vi "Dashboard Main.vi"() -> ()   [LabVIEW 2018]
uses:
  <vilib>/Utility/miscctls.llb/LVRowAndColumnTypeDef.ctl
  <vilib>/event_ctls.llb/eventvkey.ctl
  <vilib>/Rock Robotics/Network Tables/NT Read Boolean.vi
  <vilib>/Rock Robotics/Network Tables/NT Write Boolean.vi
  <vilib>/Rock Robotics/Network Tables/NT Read Numeric Array.vi
  <vilib>/Rock Robotics/WPI/Dashboard/WPI_DashboardLogging Global.vi
panel:
  in  "Camera Settings Right":T1={"Frame Rate"=30, "Compression"=30, "Size"=1, "DB Camera Config"=FALSE} {"Frame Rate" scale=1.0..30.0; "Compression" scale=100.0..-1.0; "Size" items=["640x480", "320x240", "160x120"]}
  in  "Camera Name Right":string(combo)="No Camera Selection"
  out "Camera Perf":string
  in  "Camera Settings":T1={"Frame Rate"=30, "Compression"=30, "Size"=1, "DB Camera Config"=FALSE} {"Frame Rate" scale=1.0..30.0; "Compression" scale=100.0..-1.0; "Size" items=["640x480", "320x240", "160x120"]}
  in  "TCP":refnum<k5>
  in  "Rec Mode":enum32{"Stop", "Record", "Playback"}(radio)
  out "Image Message":string="Timeout in Camera Communications"
  in  "Dashboard Tab":T2(tab)
  in  "Auto Side":bool
  out "Limelight Target State":bool
  out "Hatch Open":bool
  out "Hatch Extend":bool
  out "Cargo Piston":bool
  in  "Zero Yaw":bool
  out "Yaw":dbl
  out "Cont Yaw":dbl
  out "LowerLimit":bool
  out "UpperLimit":bool
  out "HAB Retracting limit":bool
  out "HAB Extending limit":bool
  in  "Select Auto":string(combo)="Select Autonomous ..."
  out "NT Connection":bool
  out "Mode":T3(ring)=enum."Auto Disabled"
  out "Right Camera Perf":cluster{"Bandwidth (Mbps)":dbl, "FPS":dbl}
  out "Lift Auto Position":u16(ring) items=["Cargo 1", "Hatch 1", "Cargo 2", "Hatch 2", "Cargo 3", "Hatch 3"]
  out "CargoLimit":bool
  out "Wheel Rates":T4
  out "Wheel Angles":T4
  out "Y-Velocity":dbl
  out "X-Velocity":dbl
  out "Wheel Positions":T4
  out "Lift Height":dbl
  out "Graph":cluster{cluster{"X":dbl, "Y":dbl}[]}[](graph)
  out "Positions":cluster{"X":dbl, "Y":dbl}
  out "Tree":string(tree)
  in  "Test Slider":dbl(slide) scale=0.0..100.0 scale format="%#_3g"
  in  "On/Off":bool caption="Solenoid"
  in  "Test Name":u16(ring) items=["Select the test to run..."]
  in  "Test Tree":string(tree)
  in  "Motor":cluster{"Value":dbl, "Enable":bool} {"Value" scale=-1.0..1.0 scale format="%#_3g"}
  out "Progress":T5 {"Test Progress" scale=0.0..100.0}
  in  "Rev/Fwd":cluster{"Forward":bool, "Reverse":bool}
  in  "Test Ring":u16(ring) items=["Monochrome", "Color"]
  in  "CheckList":i32(listbox)
  out "Cmd Status":string
  in  "Execute Command":bool
  in  "Command Params":string[][](table)
  in  "Command Selection":i32(listbox)
  out "Camera Image":T6(plugin-control)
  in  "Camera Name":string(combo)="No Camera Selection"
  # "HW"
  # "HW"
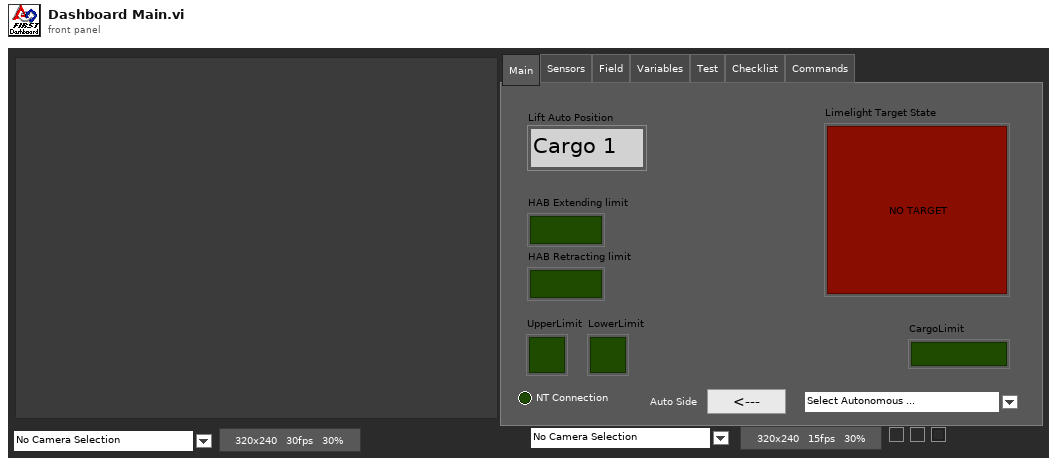
[diagram p1: front panel]
types:
  T1 = cluster{"Frame Rate":i32, "Compression":i32, "Size":u16, "DB Camera Config":bool}
  T2 = enum32{"Main", "Sensors", "Field", "Variables", "Test", "Checklist", "Commands"}
  T3 = enum8{"Tele-Op Disabled", "Tele-Op Enabled", "Auto Disabled", "Auto Enabled", "Test Disabled", "Test Enabled", "Disconnected", "No Code", "E-Stop"}
  T4 = cluster{"FrontLeft":dbl, "FrontRight":dbl, "BackLeft":dbl, "BackRight":dbl}
  T5 = cluster{"Test Progress":u8, "Test Progress Text":string}
  T6 = typedef "IMAQ Image.ctl" = refnum<image>
  T7 = cluster{"Save Path":path, "Interval (s)":dbl, "Keep":i32}
  T8 = enum32{"Drive", "Camera", "Basic", "Custom", "Test", "Commands", "Checklist", "Variables"}
  T9 = typedef "Image Type" = u32
  T10 = cluster{"IDs":cluster{"RPC field ID":u16, "Unique ID":u16}, "String":string}
  T11 = cluster{"Error Strings":string, "Disable Counts":cluster{u16, u16}, "Rail Faults":cluster{u16, u16, u16}, "Robot IP":string, "DB Mode":u8, "Event Info":cluster{"Name":string, "Type":u8, "Number":u16, "Replay":u8}}
  T12 = cluster{"Storage":cluster{"Disk Free":u64, "RAM Block":u32, "RAM free":u32}, "CPU Utilization":cluster{"CPU % ISR":sgl, "CPU % Time Crit":sgl, "CPU % Timed Str":sgl, "CPU % High":sgl, "CPU % Above":sgl, "CPU % Normal":sgl, "CPU % Low":sgl}, "CAN":cluster{"% Bus Utilization":sgl, "Bus Off Cnt":u32, "TX_FIFO Full Cnt":u32, "Receive Error Cnt":u8, "Transmit Error Cnt":u8}, "HID":cluster{"HID Outputs":u32, "Rumble Low":u16, "Rumble High":u16}[]}
  T13 = cluster{"Status bits":cluster{"Test Mode":bool, "Autonomous":bool, "Enabled":bool, "Code Start":bool, "Brownout":bool, "Reserved 2":bool, "Reserved 3":bool, "E-Stop":bool}, "Code Trace":cluster{"Disabled":bool, "TeleOp":bool, "Auto":bool, "Test":bool}, "Controller Type":enum16{"unknown", "cRIO", "roboRio"}, "Code?":enum16{"unknown", "noCode", "code"}, "Battery V":dbl}
  T14 = cluster{"Control Bits":cluster{"TestMode":bool, "Autonomous":bool, "Enabled":bool, "FMS Present":bool, bool, bool, bool, "E-Stop":bool}, "Team Station ":u8, "Countdown":sgl, "Joystick Values":cluster{"Axes":dbl[], "Buttons":bool[], "POVs":i16[]}[]}
  T15 = cluster{"Numeric":dbl, "Numeric":dbl, "Numeric":dbl, "Numeric":dbl}
  T16 = cluster{"Global Rectangle":i32[], "Contours":cluster{"Contour Type":u32, "ROI Type":u32, "Points":i32[]}[]}
  T17 = cluster{"Camera Name":string, string, "Saved DB Images Info":cluster{"Save Path":path, "Interval (s)":dbl, "Keep":i32}}
  T18 = cluster{"Camera Name Right":string, string, "Saved DB Images Info":cluster{"Save Path":path, "Interval (s)":dbl, "Keep":i32}}
  T19 = cluster{"Operation":enum16{"Update", "Clear"}, "Color Box":u32}[]
  T20 = typedef "eventvkey.ctl" = enum16{"ASCII", "Enter", "Return", "Shift", "Ctrl", "Alt", "Cmd", "Opt", "Caps", "NumLock", "Clear", "Break", "Up", "Down", "Left", "Right", "Insert", "Delete", "Home", "End", "PageUp", "PageDown", "Escape", "Help", "Pause", "ScrollLock", "F1", "F2", "F3", "F4", "F5", "F6", "F7", "F8", "F9", "F10", "F11", "F12", "F13", "F14", "F15", "F16", "F17", "F18", "F19", "F20", "F21", "F22", "F23", "F24", "Play", "VolumeUp", "VolumeDown", "Mute", "Two Byte Char"}
  T21 = cluster{"Operation":enum16{"Update", "Clear"}, "Color Box":u32}
  T22 = typedef "LVRowAndColumnTypeDef.ctl" = cluster{"Row":i32, "Column":i32}
  T23 = cluster{"Shift":bool, "Ctrl":bool, "Alt":bool, "Cmd":bool, "Opt":bool}
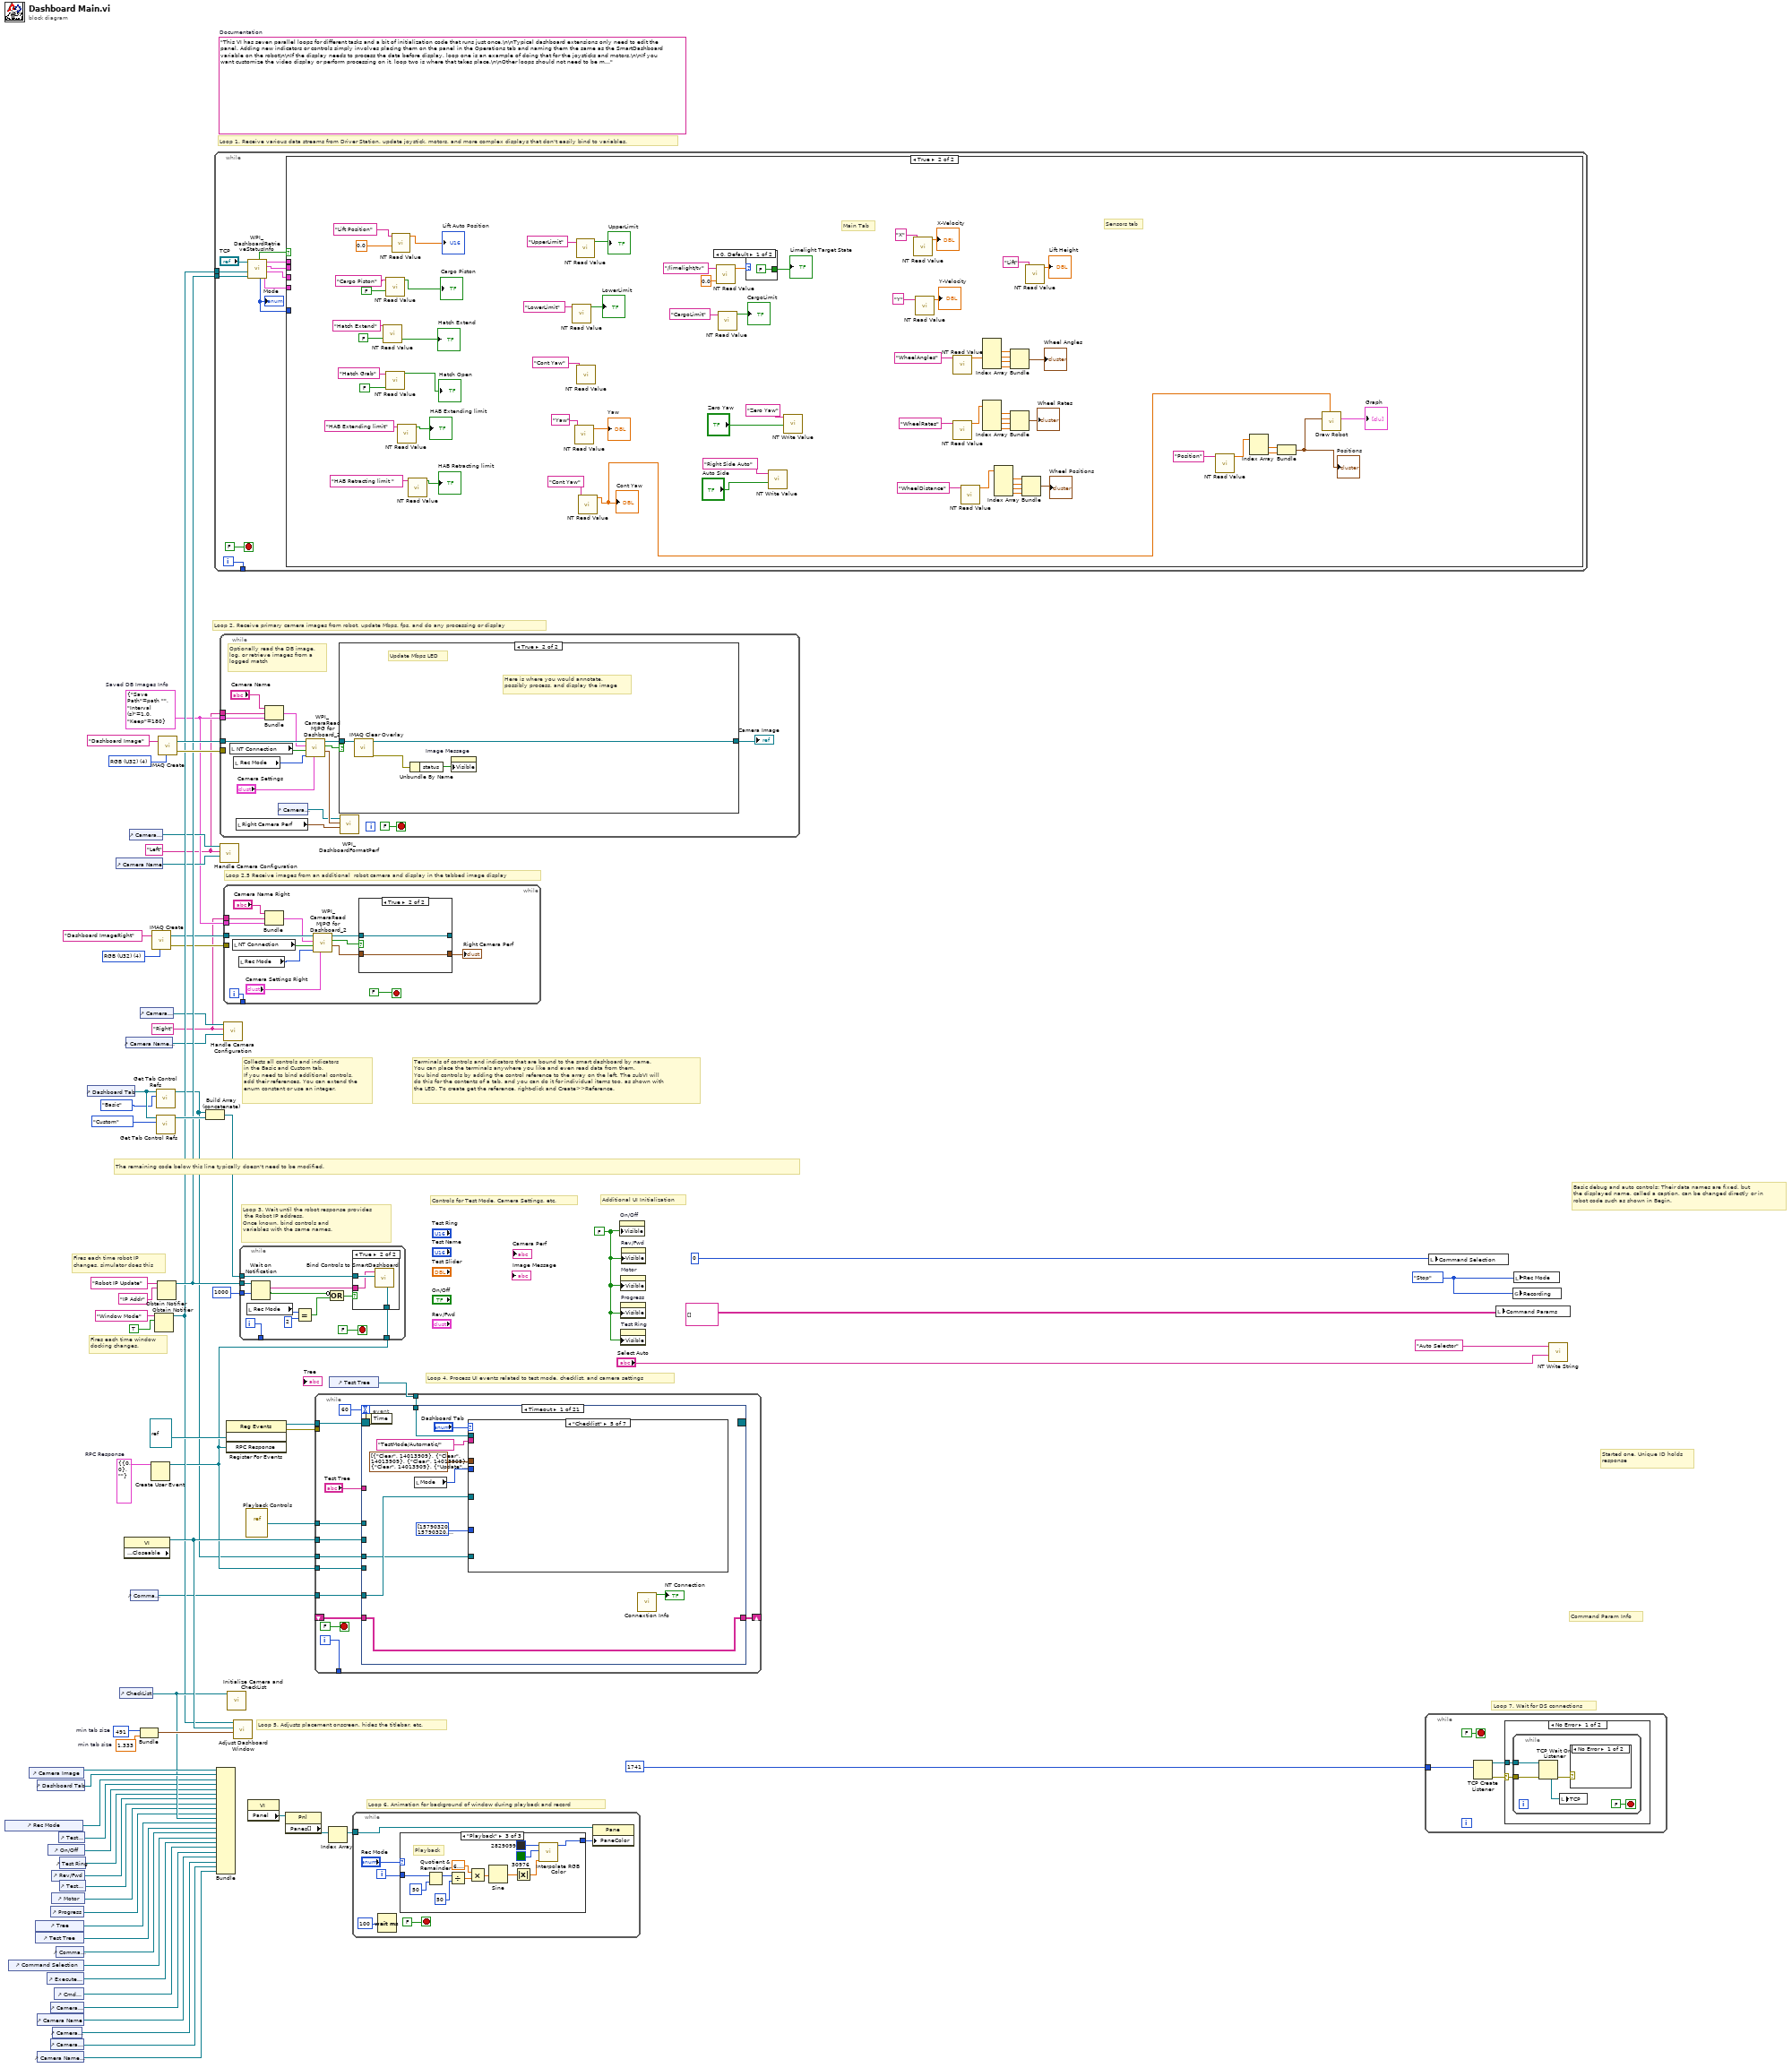
[diagram p0: block diagram]
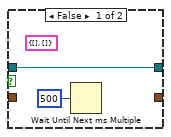
[diagram p2: hidden frame]
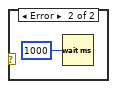
[diagram p3: hidden frame]
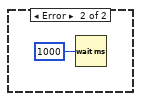
[diagram p4: hidden frame]
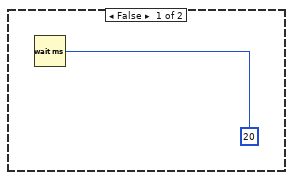
[diagram p5: hidden frame]
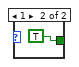
[diagram p6: hidden frame]
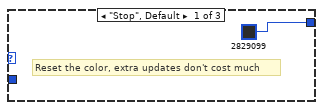
[diagram p7: hidden frame]
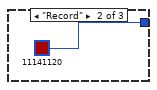
[diagram p8: hidden frame]
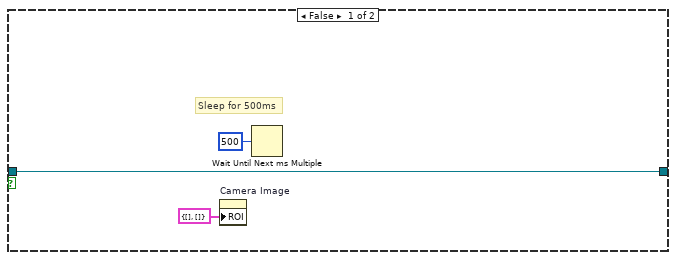
[diagram p10: hidden frame]
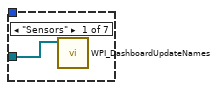
[diagram p11: hidden frame]
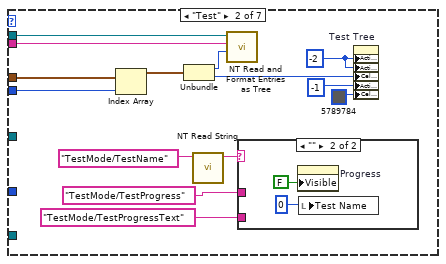
[diagram p12: hidden frame]
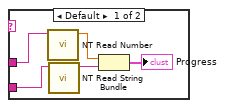
[diagram p13: hidden frame]
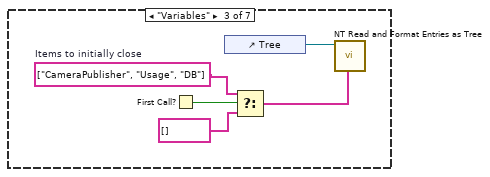
[diagram p14: hidden frame]
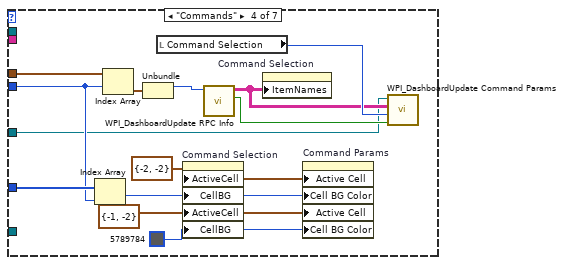
[diagram p15: hidden frame]
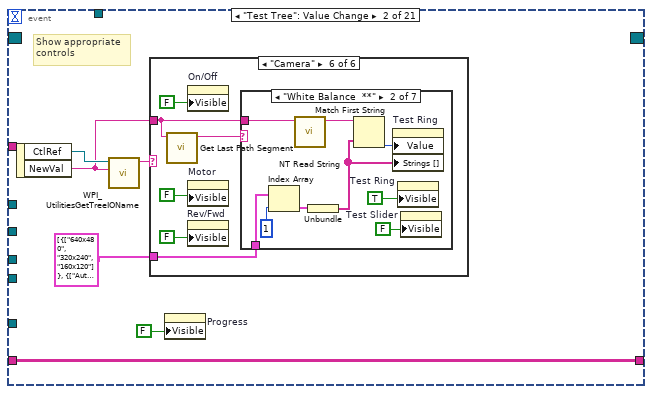
[diagram p18: hidden frame]
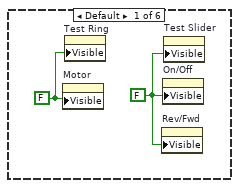
[diagram p19: hidden frame]
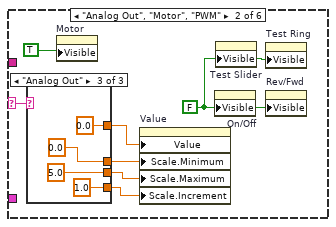
[diagram p20: hidden frame]
diagram:
  w3 = T7 {"Save Path"=path "", "Interval (s)"=1.0, "Keep"=180}  # Saved DB Images Info
  w2 = "Right"
  w1 = "Left"
  w12 = T9 4 items=["Grayscale (U8)", "Grayscale (I16)", "Grayscale (SGL)", "Complex (CSG)", "RGB (U32)", "HSL (U32)", "RGB (U64)"] ("Image Type")
  w28 = T10 {"IDs"={"RPC field ID"=0, "Unique ID"=0}, "String"=""}  # RPC Response
  w48 = 491  # min tab size
  w47 = 1.333  # min tab size
  w55 = enum32{"Stop", "Record", "Playback"}."Stop" ("Rec Mode")
  w34 = FALSE ("Visible")
  (unwired) "This VI has seven parallel loops for different tasks and a bit of initialization code that runs just once.\n\nTypical dashboard extensions only need to edit the panel. Adding new indicators or controls simply involves placing them on the panel in the Operations tab and naming them the same as the SmartDashboard variable on the robot\n\nIf the display needs to process the data before display, loop one is an example of doing that for the joysticks and motors.\n\nIf you want customize the video display or perform processing on it, loop two is where that takes place.\n\nOther loops should not need to be modified. They are pretty standard, and document the task they perform."  # Documentation
  w72 = T9 4 items=["Grayscale (U8)", "Grayscale (I16)", "Grayscale (SGL)", "Complex (CSG)", "RGB (U32)", "HSL (U32)", "RGB (U64)"] ("Image Type")
  # "Loop 2.5 Receive images from an additional  robot camera and display in the tabbed image display"
  # "Command Param Info"
  # "Started one, Unique ID holds\nresponse"
  # "Loop 7. Wait for DS connections"
  # "Basic debug and auto controls: Their data names are fixed, but\nthe displayed name, called a caption, can be changed directly or in\nrobot code such as shown in Begin."
  # "Controls for Test Mode, Camera Settings, etc."
  # "Additional UI Initialization"
  # "Loop 6. Animation for background of window during playback and record"
  # "Fires each time robot IP\nchanges, simulator does this"
  # "Fires each time window\ndocking changes."
  # "Collects all controls and indicators\nin the Basic and Custom tab.\nIf you need to bind additional controls,\nadd their references. You can extend the\nenum constant or use an integer."
  # "The remaining code below this line typically doesn't need to be modified."
  # "Loop 4. Process UI events related to test mode, checklist, and camera settings"
  # "Terminals of controls and indicators that are bound to the smart dashboard by name.\nYou can place the terminals anywhere you like and even read data from them.\nYou bind controls by adding the control reference to the array on the left. The subVI will\ndo this for the contents of a tab, and you can do it for individual items too, as shown with\nthe LED. To create get the reference, right-click and Create>>Reference."
  # "Loop 3. Wait until the robot response provides\n the Robot IP address.\nOnce known, bind controls and\nvariables with the same names."
  # "Loop 5. Adjusts placement onscreen, hides the titlebar, etc."
  # "Loop 1. Receive various data streams from Driver Station, update joystick, motors, and more complex displays that don't easily bind to variables."
  # "Loop 2. Receive primary camera images from robot, update Mbps, fps, and do any processing or display"
  n1 = control-ref of="Rec Mode"() -> (w40:refnum<vi>)
  n2 = control-ref of="Command Selection"() -> (w27:refnum<vi>)
  n3 = control-ref of="Camera Image"() -> (w50:refnum<vi>)
  n4 = control-ref of="Tree"() -> (w44:refnum<vi>)
  n5 = control-ref of="Test Tree"() -> (w43:refnum<vi>)
  n6 = control-ref of="Dashboard Tab"() -> (w49:refnum<vi>)
  n7 = control-ref of="Camera Name"() -> (w18:refnum<vi>)
  n8 = control-ref of="Camera Name Right"() -> (w6:refnum<vi>)
  n9 = control-ref of="Execute Command"() -> (w29:refnum<vi>)
  n10 = control-ref of="On/Off"() -> (w38:refnum<vi>)
  n11 = control-ref of="Progress"() -> (w35:refnum<vi>)
  n12 = control-ref of="Camera Settings"() -> (w19:refnum<vi>)
  n13 = control-ref of="Camera Settings Right"() -> (w7:refnum<vi>)
  n14 = control-ref of="Rev/Fwd"() -> (w36:refnum<vi>)
  n15 = control-ref of="Motor"() -> (w41:refnum<vi>)
  n16 = control-ref of="Camera Perf"() -> (w17:refnum<vi>)
  n17 = control-ref of="Cmd Status"() -> (w23:refnum<vi>)
  n18 = control-ref of="Command Params"() -> (w30:refnum<vi>)
  n19 = control-ref of="Test Slider"() -> (w39:refnum<vi>)
  n20 = control-ref of="Test Ring"() -> (w37:refnum<vi>)
  n21 = control-ref of="Test Name"() -> (w42:refnum<vi>)
  n22 = control-ref of="Dashboard Tab"() -> (w53:refnum<vi>)
  n23 = control-ref of="Camera Name"() -> (w20:refnum<vi>)
  n24 = control-ref of="CheckList"() -> (w45:refnum<vi>)
  n25 = property class="VI" props=["Front Panel.Closeable"]() -> (reference out=w54:refnum<vi>)  [unwired: 2 in, 2 out]
  n26 = control-ref of="Camera Name Right"() -> (w8:refnum<vi>)
  n27 = control-ref of="Camera Settings"() -> (w21:refnum<vi>)
  n28 = control-ref of="Command Params"() -> (w22:refnum<vi>)
  n29 = control-ref of="Camera Settings Right"() -> (w9:refnum<vi>)
  n30 = Bundle("min tab size"=w48, "min tab size"=w47) -> (w46:cluster{"min tab size":i32, "min tab size":dbl})  [unwired: 1 in]
  n31 = Create User Event(user event datatype=w28) -> (user event=w24:refnum<user-event>)  [unwired: 1 in, 1 out]
  n32 = call "IMAQ Create"("Image Name"="Dashboard ImageRight", "Image Type"=w12) -> ("New Image"=w11:T6, "error out"=w10:errorcluster)  [unwired: 2 in, 1 out]
  n33 = Obtain Notifier(name (unnamed)="Window Mode", notification data type=TRUE) -> (notifier out=w32:refnum<notifier>)  [unwired: 2 in, 2 out]
  n34 = call <vilib>:"Get Tab Control Refs.vi"("Page Index"=T8."Basic" ("Dashboard Tab"), "TabControl in"=w53) -> ("ControlsOnPage"=w16:refnum<vi>[])  [unwired: 9 in]
  n35 = call <vilib>:"Get Tab Control Refs.vi"("Page Index"=T8."Custom" ("Dashboard Tab"), "TabControl in"=w53) -> ("ControlsOnPage"=w52:refnum<vi>[])  [unwired: 9 in]
  n36 = Obtain Notifier(name (unnamed)="Robot IP Update", notification data type="IP Addr" ("name (unnamed)")) -> (notifier out=w33:refnum<notifier>)  [unwired: 2 in, 2 out]
  n37 = call "IMAQ Create"("Image Name"="Dashboard Image", "Image Type"=w72) -> ("New Image"=w70:T6, "error out"=w69:errorcluster)  [unwired: 2 in, 1 out]
  n38 = Build Array (concatenate)(w16, w52) -> (w51:refnum<vi>[])
  n39 = while {
    tunnel: [w82] -> _
    tunnel: w33 -> [w80]
    tunnel: w32 -> [w77]
    i -> [w82]
    stop <- FALSE stop-if-true
    n40 = call <vilib>:"WPI_DashboardRetrieveStatusInfo.vi"("Binding Refnum"=w80, "Window Mode Notifier"=w77, "TCP Cnx"="TCP") -> ("Power and Errors"=w74:T11, "Robot Metrics"=w73:T12, "Status Info"=w75:T13, "Control Info"=w76:T14, "Robot Mode"=w79:T3, "Process?"=w81:bool)  [unwired: 3 in]
    "Mode" <- w79
    n41 = case shown="True" w81 {
      tunnel: w79 -> [_ _]
      tunnel: w76 -> [_ _]
      tunnel: w75 -> [_ _]
      tunnel: w74 -> [_ _]
      tunnel: w73 -> [_ _]
      frame False {
        n42 = Wait (ms)(milliseconds to wait=u32 20) -> ()  [unwired: 1 out]
      }
      frame True {
        # "Sensors tab"
        # "Main Tab"
        n43 = call-poly <vilib>:"NT Read Value.vi"("Default Value"=FALSE, "Name"="Hatch Extend") -> ("Boolean"=→"Hatch Extend":bool)  [unwired: 8 in, 1 out]
        n44 = call-poly <vilib>:"NT Read Value.vi"("Default Value"=FALSE, "Name"="Cargo Piston") -> ("Boolean"=→"Cargo Piston":bool)  [unwired: 8 in, 1 out]
        n45 = call-poly <vilib>:"NT Read Value.vi"("Default Value"=FALSE, "Name"="Hatch Grab") -> ("Boolean"=→"Hatch Open":bool)  [unwired: 8 in, 1 out]
        n46 = call-poly <vilib>:"NT Read Value.vi"("Default Value"=0.0, "Name"="Lift Position") -> ("Numeric"=→"Lift Auto Position":dbl)  [unwired: 8 in, 1 out]
        n47 = call-poly <vilib>:"NT Read Value.vi"("Name"="HAB Extending limit") -> ("Boolean"=→"HAB Extending limit":bool)  [unwired: 9 in, 1 out]
        n48 = call-poly <vilib>:"NT Read Value.vi"("Name"="HAB Retracting limit ") -> ("Boolean"=→"HAB Retracting limit":bool)  [unwired: 9 in, 1 out]
        n49 = call-poly <vilib>:"NT Read Value.vi"("Name"="LowerLimit") -> ("Boolean"=→"LowerLimit":bool)  [unwired: 9 in, 1 out]
        n50 = call-poly <vilib>:"NT Read Value.vi"("Name"="Yaw") -> ("Numeric"=→"Yaw":dbl)  [unwired: 9 in, 1 out]
        n51 = call-poly <vilib>:"NT Read Value.vi"("Name"="UpperLimit") -> ("Boolean"=→"UpperLimit":bool)  [unwired: 9 in, 1 out]
        n52 = call-poly <vilib>:"NT Read Value.vi"("Name"="Cont Yaw") -> ()  [unwired: 9 in, 2 out]
        n53 = call-poly <vilib>:"NT Read Value.vi"("Name"="Cont Yaw") -> ("Numeric"=w85:dbl)  [unwired: 9 in, 1 out]
        "Cont Yaw" <- w85
        n54 = call-poly <vilib>:"NT Read Value.vi"("Default Value"=0.0, "Name"="/limelight/tv") -> ("Numeric"=w120:dbl)  [unwired: 8 in, 1 out]
        n55 = call-poly <vilib>:"NT Read Value.vi"("Name"="CargoLimit") -> ("Boolean"=→"CargoLimit":bool)  [unwired: 9 in, 1 out]
        n56 = case shown="0, Default" w120 {
          tunnel: [FALSE TRUE] -> w119
          frame 0, Default {
          }
          frame 1 {
          }
        }
        "Limelight Target State" <- w119
        n57 = call-poly <vilib>:"NT Write Value.vi"("Boolean"="Auto Side", "Name"="Right Side Auto") -> ()  [unwired: 9 in, 1 out]
        n58 = call-poly <vilib>:"NT Write Value.vi"("Boolean"="Zero Yaw", "Name"="Zero Yaw") -> ()  [unwired: 9 in, 1 out]
        n59 = call-poly <vilib>:"NT Read Value.vi"("Name"="X") -> ("Numeric"=→"X-Velocity":dbl)  [unwired: 9 in, 1 out]
        n60 = call-poly <vilib>:"NT Read Value.vi"("Name"="Y") -> ("Numeric"=→"Y-Velocity":dbl)  [unwired: 9 in, 1 out]
        n61 = call-poly <vilib>:"NT Read Value.vi"("Name"="WheelAngles") -> ("Numeric Array"=w117:dbl[])  [unwired: 9 in, 1 out]
        n62 = call-poly <vilib>:"NT Read Value.vi"("Name"="WheelRates") -> ("Numeric Array"=w107:dbl[])  [unwired: 9 in, 1 out]
        n63 = call-poly <vilib>:"NT Read Value.vi"("Name"="WheelDistance") -> ("Numeric Array"=w102:dbl[])  [unwired: 9 in, 1 out]
        n64 = Index Array(array=w117) -> (element #1=w116:dbl, element #2=w115:dbl, element #3=w114:dbl, element #4=w113:dbl)  [unwired: 4 in]
        n65 = Index Array(array=w107) -> (element #1=w108:dbl, element #2=w109:dbl, element #3=w110:dbl, element #4=w111:dbl)  [unwired: 4 in]
        n66 = Index Array(array=w102) -> (element #1=w101:dbl, element #2=w100:dbl, element #3=w99:dbl, element #4=w98:dbl)  [unwired: 4 in]
        n67 = Bundle("Numeric"=w116, "Numeric"=w115, "Numeric"=w114, "Numeric"=w113) -> (→"Wheel Angles":T15)  [unwired: 1 in]
        n68 = Bundle("Numeric"=w108, "Numeric"=w109, "Numeric"=w110, "Numeric"=w111) -> (→"Wheel Rates":T15)  [unwired: 1 in]
        n69 = Bundle("Numeric"=w101, "Numeric"=w100, "Numeric"=w99, "Numeric"=w98) -> (→"Wheel Positions":T15)  [unwired: 1 in]
        n70 = call-poly <vilib>:"NT Read Value.vi"("Name"="Lift") -> ("Numeric"=→"Lift Height":dbl)  [unwired: 9 in, 1 out]
        n71 = call-poly <vilib>:"NT Read Value.vi"("Name"="Position") -> ("Numeric Array"=w89:dbl[])  [unwired: 9 in, 1 out]
        n72 = Index Array(array=w89) -> (element #1=w90:dbl, element #2=w91:dbl)  [unwired: 2 in]
        n73 = Bundle("Numeric"=w90, "Numeric"=w91) -> (w86:cluster{"Numeric":dbl, "Numeric":dbl})  [unwired: 1 in]
        "Positions" <- w86
        n74 = call "Draw Robot.vi"("Gyro"=w85, "XY"=w86) -> ("Graph 2"=→"Graph":cluster{cluster{"X":dbl, "Y":dbl}[]}[])  [unwired: 9 in]
      }
    }
  }
  n75 = Bundle("Camera Image"=w50, "Dashboard Tab"=w49, "Rec Mode"=w40, "Test Slider"=w39, "On/Off"=w38, "Test Ring"=w37, "Rev/Fwd"=w36, "Test Name"=w42, "Motor"=w41, "Progress"=w35, "CheckList"=w45, "Tree"=w44, "Test Tree"=w43, "Command Params"=w30, "Command Selection"=w27, "Execute Command"=w29, "Cmd Status"=w23, "Camera Settings"=w19, "Camera Name"=w18, "Camera Perf"=w17, "Camera Settings Right"=w7, "Camera Name Right"=w6) -> ()  [unwired: 1 in, 1 out]
  n76 = call "Handle Camera Configuration.vi"("CameraNameRef"=w20, "Display Name"=w1, "ClusterRef"=w21) -> ()  [unwired: 9 in]
  n77 = while {
    tunnel: w70 -> [w168]
    tunnel: w69 -> [_]
    tunnel: w3 -> [w161]
    tunnel: w1 -> [w158]
    stop <- FALSE stop-if-true
    # "Optionally read the DB image,\nlog, or retrieve images from a\nlogged match"
    n78 = local read "NT Connection"() -> (w162:bool)
    n79 = local read "Rec Mode"() -> (w165:enum32{"Stop", "Record", "Playback"})
    n80 = local read "Right Camera Perf"() -> (w156:cluster{"Bandwidth (Mbps)":dbl, "FPS":dbl})
    n81 = Bundle("Camera Name"="Camera Name", w158, "Saved DB Images Info"=w161) -> (w160:T17)  [unwired: 1 in]
    n82 = control-ref of="Camera Perf"() -> (w155:refnum<vi>)
    n83 = call <vilib>:"WPI_CameraRead MJPG for Dashboard_2.vi"("Camera Settings"="Camera Settings", "Rec Mode"=w165, "NT Connection"=w162, "Capture Info"=w160, "Image in"=w168) -> ("perf info"=w157:cluster{"Bandwidth (Mbps)":dbl, "fps":dbl}, "Active"=w166:bool, "Image\\ out"=w167:T6)  [unwired: 4 in]
    n84 = case shown="True" w166 {
      tunnel: w167 -> [w171 w174]
      tunnel: [w171 w173] -> w163
      frame False {
        # "Sleep for 500ms"
        n85 = property on="Camera Image" class="ImageControl"("ROI"=T16 {"Global Rectangle"=[], "Contours"=[]}) -> ()  [unwired: 2 in, 2 out]
        n86 = Wait Until Next ms Multiple(millisecond multiple=u32 500) -> ()  [unwired: 1 out]
      }
      frame True {
        # "Here is where you would annotate,\npossibly process, and display the image"
        # "Update Mbps LED"
        n87 = call "IMAQ Clear Overlay"("Image"=w174) -> ("error out"=w175:errorcluster, "Image Out"=w173:T6)  [unwired: 2 in, 7 out]
        n88 = Unbundle By Name(w175) -> ("status"=w176:bool)
        n89 = property on="Image Message" class="Str"("Visible"=w176) -> ()  [unwired: 2 in, 2 out]
      }
    }
    "Camera Image" <- w163
    n90 = call <vilib>:"WPI_DashboardFormatPerf.vi"("Right Camera Perf"=w156, "Performance"=w157, "String in"=w155) -> ()  [unwired: 9 in]
  }
  n91 = call "Handle Camera Configuration.vi"("CameraNameRef"=w8, "Display Name"=w2, "ClusterRef"=w9) -> ()  [unwired: 9 in]
  n92 = while {
    tunnel: w11 -> [w190]
    tunnel: w10 -> [_]
    tunnel: [w185] -> _
    tunnel: w3 -> [w182]
    tunnel: w2 -> [w179]
    i -> [w185]
    stop <- FALSE stop-if-true
    n93 = local read "NT Connection"() -> (w183:bool)
    n94 = local read "Rec Mode"() -> (w189:enum32{"Stop", "Record", "Playback"})
    n95 = Bundle("Camera Name Right"="Camera Name Right", w179, "Saved DB Images Info"=w182) -> (w181:T18)  [unwired: 1 in]
    n96 = call <vilib>:"WPI_CameraRead MJPG for Dashboard_2.vi"("Camera Settings"="Camera Settings Right", "Rec Mode"=w189, "NT Connection"=w183, "Capture Info"=w181, "Image in"=w190) -> ("perf info"=w177:cluster{"Bandwidth (Mbps)":dbl, "fps":dbl}, "Active"=w184:bool, "Image\\ out"=w187:T6)  [unwired: 4 in]
    n97 = case shown="True" w184 {
      tunnel: w187 -> [w191 w194]
      tunnel: [w191 w194] -> _
      tunnel: [_ w193] -> w178
      tunnel: w177 -> [_ w193]
      frame False {
        (unwired) T16 {"Global Rectangle"=[], "Contours"=[]} ("ROI")
        n98 = Wait Until Next ms Multiple(millisecond multiple=u32 500) -> ()  [unwired: 1 out]
      }
      frame True {
      }
    }
    "Right Camera Perf" <- w178
  }
  n99 = register-events(refnum<vi> refnum, w24) -> (reference out=w59:refnum<event-registration>, error out=w58:errorcluster)  [unwired: 2 in]
  n100 = call "Initialize Camera and CheckList.vi"("ListBox in"=w45) -> ()  [unwired: 11 in]
  n101 = call "Adjust Dashboard Window.vi"("Size Constraints"=w46, "VI"=w54, "WIn Mode"=w32) -> ()  [unwired: 9 in]
  n102 = while {
    tunnel: w51 -> [w206]
    tunnel: w33 -> [w204]
    tunnel: [w202] -> _
    tunnel: u32 1000 ("milliseconds to wait") -> [w201]
    tunnel: w24 -> [w195]
    i -> [w202]
    stop <- FALSE stop-if-true
    n103 = local read "Rec Mode"() -> (w197:enum32{"Stop", "Record", "Playback"})
    n104 = Wait on Notification(notifier=w204, timeout in ms (-1)=w201) -> (notification=w203:string, timed out?=w199:bool)  [unwired: 2 in, 2 out]
    n105 = Equal?(x=w197, y=u16 2 ("Rec Mode")) -> (x = y?=w198:bool)
    n106 = Compound Arithmetic op=OR(invert w199, w198) -> (w200:bool)
    n107 = case shown="True" w200 {
      tunnel: w206 -> [_ w209]
      tunnel: w203 -> [_ w208]
      tunnel: w195 -> [_ w207]
      frame False {
      }
      frame True {
        n108 = call <vilib>:"Bind Controls to SmartDashboard.vi"("RPC ref"=w207, "Bound Control Refs"=w209, "Server IP Address"=w208) -> ()  [unwired: 9 in]
      }
    }
  }
  n109 = vi-ref "Playback Controls.vi"() -> (w60:refnum<vi>)
  n110 = property class="VI"() -> ("Panel"=w62:refnum<vi>)  [unwired: 2 in, 2 out]
  n111 = property class="Pnl"(reference=w62) -> ("Panes[]"=w63:refnum<vi>[])  [unwired: 1 in, 2 out]
  n112 = Index Array(array=w63) -> (element=w61:refnum<vi>)  [unwired: 1 in]
  n113 = control-ref of="Test Tree"() -> (w64:refnum<vi>)
  n114 = while {
    tunnel: [w219] -> _
    tunnel: w64 -> [w218]
    tunnel: w60 -> [w217]
    tunnel: w59 -> [w216]
    tunnel: w58 -> [_]
    tunnel: w54 -> [w215]
    tunnel: w24 -> [w214]
    tunnel: w22 -> [w213]
    shift-right: [w212] -> _
    shift-left: _ -> [w211]
    tunnel: w16 -> [w210]
    i -> [w219]
    stop <- FALSE stop-if-true
    n115 = event shown="[0] Timeout" {
      selector: w216 -> [_ _ _ _ _ _ _ _ _ _ _ _ _ _ _ _ _ _ _ _ _]
      dyn-events: [_ _ _ _ _ _ _ _ _ _ _ _ _ _ _ _ w477 _ _ _ _] -> _
      timeout: u32 60 ("milliseconds to wait") -> [_ _ _ _ _ _ _ _ _ _ _ _ _ _ _ _ _ _ _ _ _]
      tunnel: w218 -> [w231 _ _ _ _ _ _ _ _ _ _ _ _ _ _ _ _ _ _ _ _]
      tunnel: "Test Tree" -> [_ _ _ _ _ _ _ _ _ _ _ w446 w454 w456 w460 w468 _ _ _ _ _]
      tunnel: w217 -> [_ _ _ _ _ _ _ _ _ _ _ _ _ _ _ _ w479 _ w495 _ _]
      tunnel: w215 -> [_ _ _ _ _ _ _ _ _ _ _ _ _ _ _ _ w475 _ _ _ _]
      tunnel: w214 -> [_ _ _ _ _ _ _ _ _ _ _ _ _ _ _ _ w473 _ _ _ _]
      tunnel: w213 -> [w226 _ _ _ _ _ w397 _ _ _ _ _ _ _ _ _ _ _ _ _ _]
      tunnel: [w225 w274 w376 w381 w390 w394 w395 w404 w414 w421 w433 w445 w452 w455 w459 w467 w472 w490 w492 w496 w509] -> w212
      tunnel: w211 -> [w225 w274 w376 w381 w390 w394 w395 _ _ w421 w433 w445 w452 w455 w459 w467 w472 w490 w492 w496 w509]
      tunnel: w210 -> [w223 _ _ _ _ _ _ _ _ _ _ _ _ _ _ _ _ _ _ _ _]
      event Timeout {
        n116 = event-data() -> ()  [unwired: 1 in, 1 out]
        n117 = local read "Mode"() -> (w228:T3)
        n118 = case shown="\"Checklist\"" "Dashboard Tab" {
          tunnel: w231 -> [_ w247 _ _ _ _ _]
          tunnel: "TestMode/Automatic/" ("Name Pattern") -> [_ w246 _ _ _ _ _]
          tunnel: T19 [{"Operation"=enum."Clear", "Color Box"=14013909}, {"Operation"=enum."Clear", "Color Box"=14013909}, {"Operation"=enum."Clear", "Color Box"=14013909}, {"Operation"=enum."Clear", "Color Box"=14013909}, {"Operation"=enum."Update", "Color Box"=14013909}, {"Operation"=enum."Update", "Color Box"=16777215}, {"Operation"=enum."Clear", "Color Box"=14013909}, {"Operation"=enum."Clear", "Color Box"=14013909}, {"Operation"=enum."Clear", "Color Box"=14013909}] -> [_ w239 _ w267 _ _ _]
          tunnel: w228 -> [_ w238 _ w266 _ _ _]
          tunnel: u32[] [15790320, 15790320, 15790320, 15790320, 16777215, 16777215, 15790320, 15790320, 15790320] -> [_ _ _ w272 _ _ _]
          tunnel: w226 -> [_ _ _ w260 _ _ _]
          tunnel: w223 -> [w233 _ _ _ _ _ _]
          frame "Sensors" {
            n119 = call <vilib>:"WPI_DashboardUpdateNames.vi"("Controls on Tab"=w233) -> ()  [unwired: 11 in]
          }
          frame "Test" {
            w245 = -2 ("Active Item:Row Number")
            n120 = Index Array(array=w239, index=w238) -> (element=w240:T21)
            n121 = Unbundle(w240) -> ("Operation"=w241:enum16{"Update", "Clear"}, "Color Box"=w242:u32)
            n122 = call <vilib>:"NT Read String.vi"("Name"="TestMode/TestName") -> ("String"=w236:string)  [unwired: 9 in, 1 out]
            n123 = call <vilib>:"NT Read and Format Entries as Tree.vi"("Operation"=w241, "Name Pattern"=w246, "Tree Refnum"=w247) -> ()  [unwired: 7 in, 2 out]
            n124 = case shown="\"\"" w236 {
              tunnel: "TestMode/TestProgress" ("Name") -> [w249 _]
              tunnel: "TestMode/TestProgressText" ("Name") -> [w248 _]
              frame Default {
                n125 = call <vilib>:"NT Read Number.vi"("Name"=w249) -> ("Numeric"=w250:dbl)  [unwired: 9 in, 1 out]
                n126 = call <vilib>:"NT Read String.vi"("Name"=w248) -> ("String"=w251:string)  [unwired: 9 in, 1 out]
                n127 = Bundle("Numeric"=w250, "String"=w251) -> (→"Progress":cluster{"Numeric":dbl, "String":string})  [unwired: 1 in]
              }
              frame "" {
                n128 = property on="Progress" class="Clust (strict)"("Visible"=FALSE) -> ()  [unwired: 2 in, 2 out]
                n129 = local write "Test Name"(u16 0) -> ()
              }
            }
            n130 = property on="Test Tree" class="Tree (strict)"("Active Item Row Number"=w245, "ActiveColNum"=w245, "CellBG"=w242, "Active Item Row Number"=-1 ("Active Item:Row Number"), "CellBG"=u32 5789784 ("Color Box")) -> ()  [unwired: 2 in, 2 out]
          }
          frame "Variables" {
            w257 = string[] ["CameraPublisher", "Usage", "DB"]  # Items to initially close
            n131 = First Call?() -> (First Call?: T/F=w258:bool)
            n132 = control-ref of="Tree"() -> (w259:refnum<vi>)
            n133 = Select(t=w257, s=w258, f=string[] []) -> (s? t:f=w255:string[])
            n134 = call <vilib>:"NT Read and Format Entries as Tree.vi"("Tags to  Close"=w255, "Tree Refnum"=w259) -> ()  [unwired: 8 in, 2 out]
          }
          frame "Commands" {
            w268 = u32 5789784 ("Color Box")
            w269 = T22 {"Row"=-1, "Column"=-2} ("Active Cell:Active Cell")
            w271 = T22 {"Row"=-2, "Column"=-2} ("Active Cell:Active Cell")
            n135 = Index Array(array=w272, index=w266) -> (element=w270:u32)
            n136 = Index Array(array=w267, index=w266) -> (element=w265:T21)
            n137 = Unbundle(w265) -> ("Operation"=w264:enum16{"Update", "Clear"})  [unwired: 1 out]
            n138 = local read "Command Selection"() -> (w263:i32)
            n139 = property on="Command Selection" class="MCListbox (strict)"("ActiveCell"=w271, "CellBG"=w270, "ActiveCell"=w269, "CellBG"=w268) -> ()  [unwired: 2 in, 2 out]
            n140 = call <vilib>:"WPI_DashboardUpdate RPC Info.vi"("Operation"=w264) -> ("update"=w262:bool, "commands"=w261:string[][])  [unwired: 9 in]
            n141 = property on="Command Selection" class="MCListbox (strict)"("ItemNames"=w261) -> ()  [unwired: 2 in, 2 out]
            n142 = property on="Command Params" class="Tbl (strict)"("Active Cell"=w271, "Cell BG Color"=w270, "Active Cell"=w269, "Cell BG Color"=w268) -> ()  [unwired: 2 in, 2 out]
            n143 = call <vilib>:"WPI_DashboardUpdate Command Params.vi"("Update"=w262, "NewVal"=w263, "Commands"=w261, "Param Tbl"=w260) -> ()  [unwired: 7 in, 1 out]
          }
          frame "Checklist" {
          }
          frame "Main" {
          }
          frame "Field" {
          }
        }
        n144 = call <vilib>:"Connextion Info.vi"() -> ("Connected"=→"NT Connection":bool)  [unwired: 10 in, 1 out]
      }
      event "Test Tree": Value Change {
        # "Show appropriate\ncontrols"
        n145 = event-data() -> ("CtlRef"=w277:refnum<vi>, "NewVal"=w275:string)  [unwired: 1 in]
        n146 = call <vilib>:"WPI_UtilitiesGetTreeIOName.vi"("NewVal"=w275, "TreeControl in"=w277) -> ("I/O Name"=w278:string)  [unwired: 9 in]
        n147 = case shown="\"Camera\"" w278 {
          selector: w278 -> [_ w285 _ w307 w316 _]
          tunnel: w275 -> [_ _ w304 w306 _ w323]
          tunnel: cluster{string[]}[] [{["640x480", "320x240", "160x120"]}, {["Auto", "Fixed indoor", "Fixed outdoor 1", "Fixed outdoor 2", "Fixed fluorescent 1", "Fixed fluorescent 2", "Hold current"]}, {["Auto", "Flicker-free 50 Hz", "Flicker-free 60 Hz", "Hold current"]}, {["None", "Prioritize frame rate", "Prioritize image quality"]}, {["Monochrome", "Color"]}] -> [_ _ _ _ _ w322]
          frame Default {
            w280 = FALSE ("Visible")
            w279 = FALSE ("Visible")
            n148 = property on="Motor" class="Clust (strict)"("Visible"=w279) -> ()  [unwired: 2 in, 2 out]
            n149 = property on="Test Ring" class="Ring (strict)"("Visible"=w279) -> ()  [unwired: 2 in, 2 out]
            n150 = property on="Rev/Fwd" class="Clust (strict)"("Visible"=w280) -> ()  [unwired: 2 in, 2 out]
            n151 = property on="On/Off" class="Bool (strict)"("Visible"=w280) -> ()  [unwired: 2 in, 2 out]
            n152 = property on="Test Slider" class="Slide (strict)"("Visible"=w280) -> ()  [unwired: 2 in, 2 out]
          }
          frame "Analog Out", "Motor", "PWM" {
            w286 = FALSE ("Visible")
            n153 = case shown="\"Analog Out\"" w285 {
              tunnel: [1.0 ("Value") -1.0 ("Value") 0.0 ("Value")] -> w284
              tunnel: [255.0 ("Value") 1.0 ("Value") 5.0 ("Value")] -> w283
              tunnel: [128.0 ("Value") 0.0 ("Value") 0.0 ("Value")] -> w282
              tunnel: [64.0 ("Value") 0.5 ("Value") 1.0 ("Value")] -> w281
              frame "PWM" {
              }
              frame "Motor", Default {
              }
              frame "Analog Out" {
              }
            }
            n154 = property on="Motor" class="Clust (strict)"("Visible"=TRUE) -> ()  [unwired: 2 in, 2 out]
            n155 = property on="Value" class="Slide (strict)"("Value"=w282, "Scale.Minimum"=w284, "Scale.Maximum"=w283, "Scale.Increment"=w281) -> ()  [unwired: 2 in, 2 out]
            n156 = property on="On/Off" class="Bool (strict)"("Visible"=w286) -> ()  [unwired: 2 in, 2 out]
            n157 = property on="Test Slider" class="Slide (strict)"("Visible"=w286) -> ()  [unwired: 2 in, 2 out]
            n158 = property on="Test Ring" class="Ring (strict)"("Visible"=w286) -> ()  [unwired: 2 in, 2 out]
            n159 = property on="Rev/Fwd" class="Clust (strict)"("Visible"=w286) -> ()  [unwired: 2 in, 2 out]
          }
          frame "Servo" {
            w302 = FALSE ("Visible")
            n160 = call <vilib>:"NT Read Number.vi"("Name"=w304) -> ("Numeric"=w303:dbl)  [unwired: 9 in, 1 out]
            n161 = property on="Test Slider" class="Slide (strict)"("Visible"=TRUE, "Scale.Maximum"=170.0 ("Scale.Range:Maximum")) -> ()  [unwired: 2 in, 2 out]
            n162 = local write "Test Slider"(w303) -> ()
            n163 = property on="Motor" class="Clust (strict)"("Visible"=w302) -> ()  [unwired: 2 in, 2 out]
            n164 = property on="Rev/Fwd" class="Clust (strict)"("Visible"=w302) -> ()  [unwired: 2 in, 2 out]
            n165 = property on="On/Off" class="Bool (strict)"("Visible"=w302) -> ()  [unwired: 2 in, 2 out]
            n166 = property on="Test Ring" class="Ring (strict)"("Visible"=w302) -> ()  [unwired: 2 in, 2 out]
          }
          frame "Relay", "Solenoid" {
            w305 = FALSE ("Visible")
            n167 = property on="Motor" class="Clust (strict)"("Visible"=w305) -> ()  [unwired: 2 in, 2 out]
            n168 = property on="Test Slider" class="Slide (strict)"("Visible"=w305) -> ()  [unwired: 2 in, 2 out]
            n169 = Search and Replace String(input string=w306, search string="/Value  **", replace string="/Direction") -> (result string=w312:string)  [unwired: 5 in, 3 out]
            n170 = property on="Test Ring" class="Ring (strict)"("Visible"=w305) -> ()  [unwired: 2 in, 2 out]
            n171 = call <vilib>:"NT Read String.vi"("Name"=w312) -> ("String"=w310:string)  [unwired: 9 in, 1 out]
            n172 = Equal?(x="Both directions", y=w310) -> (x = y?=w308:bool)
            n173 = Not(x=w308) -> (.not. x?=w309:bool)
            n174 = property on="Rev/Fwd" class="Clust (strict)"("Visible"=w308) -> ()  [unwired: 2 in, 2 out]
            n175 = property on="On/Off" class="Bool (strict)"("Visible"=w309, "Caption.Text"=w307) -> ()  [unwired: 2 in, 2 out]
          }
          frame "Compressor", "Digital Out" {
            w315 = FALSE ("Visible")
            # "Get direction and finish"
            n176 = property on="Motor" class="Clust (strict)"("Visible"=w315) -> ()  [unwired: 2 in, 2 out]
            n177 = property on="Test Slider" class="Slide (strict)"("Visible"=w315) -> ()  [unwired: 2 in, 2 out]
            n178 = property on="Test Ring" class="Ring (strict)"("Visible"=w315) -> ()  [unwired: 2 in, 2 out]
            n179 = property on="On/Off" class="Bool (strict)"("Visible"=TRUE, "Caption.Text"=w316) -> ()  [unwired: 2 in, 2 out]
            n180 = property on="Rev/Fwd" class="Clust (strict)"("Visible"=FALSE) -> ()  [unwired: 2 in, 2 out]
          }
          frame "Camera" {
            n181 = call <vilib>:"Get Last Path Segment.vi"("String in"=w323) -> ("String out"=w324:string)  [unwired: 10 in]
            n182 = property on="On/Off" class="Bool (strict)"("Visible"=FALSE) -> ()  [unwired: 2 in, 2 out]
            n183 = property on="Motor" class="Clust (strict)"("Visible"=FALSE) -> ()  [unwired: 2 in, 2 out]
            n184 = property on="Rev/Fwd" class="Clust (strict)"("Visible"=FALSE) -> ()  [unwired: 2 in, 2 out]
            n185 = case shown="\"White Balance  **\"" w324 {
              tunnel: w323 -> [w330 w339 w348 w357 w366 _ w372]
              tunnel: w322 -> [w328 w336 w345 w354 w363 _ _]
              frame "Size  **" {
                n186 = Index Array(array=w328) -> (element=w327:cluster{string[]})  [unwired: 1 in]
                n187 = call <vilib>:"NT Read String.vi"("Name"=w330) -> ("String"=w329:string)  [unwired: 9 in, 1 out]
                n188 = Unbundle(w327) -> (w325:string[])
                n189 = Match First String(2:w325, 3:w329) -> (0:w326:i32)  [unwired: 1 out]
                n190 = property on="Test Ring" class="Ring (strict)"("Value"=w326, "Strings []"=w325) -> ()  [unwired: 2 in, 2 out]
                n191 = property on="Test Ring" class="Ring (strict)"("Visible"=TRUE) -> ()  [unwired: 2 in, 2 out]
                n192 = property on="Test Slider" class="Slide (strict)"("Visible"=FALSE) -> ()  [unwired: 2 in, 2 out]
              }
              frame "White Balance  **" {
                n193 = Index Array(array=w336, index=1) -> (element=w337:cluster{string[]})
                n194 = call <vilib>:"NT Read String.vi"("Name"=w339) -> ("String"=w338:string)  [unwired: 9 in, 1 out]
                n195 = Unbundle(w337) -> (w334:string[])
                n196 = Match First String(2:w334, 3:w338) -> (0:w333:i32)  [unwired: 1 out]
                n197 = property on="Test Ring" class="Ring (strict)"("Value"=w333, "Strings []"=w334) -> ()  [unwired: 2 in, 2 out]
                n198 = property on="Test Ring" class="Ring (strict)"("Visible"=TRUE) -> ()  [unwired: 2 in, 2 out]
                n199 = property on="Test Slider" class="Slide (strict)"("Visible"=FALSE) -> ()  [unwired: 2 in, 2 out]
              }
              frame "Exposure  **" {
                n200 = Index Array(array=w345, index=2) -> (element=w346:cluster{string[]})
                n201 = call <vilib>:"NT Read String.vi"("Name"=w348) -> ("String"=w347:string)  [unwired: 9 in, 1 out]
                n202 = Unbundle(w346) -> (w342:string[])
                n203 = Match First String(2:w342, 3:w347) -> (0:w343:i32)  [unwired: 1 out]
                n204 = property on="Test Ring" class="Ring (strict)"("Value"=w343, "Strings []"=w342) -> ()  [unwired: 2 in, 2 out]
                n205 = property on="Test Ring" class="Ring (strict)"("Visible"=TRUE) -> ()  [unwired: 2 in, 2 out]
                n206 = property on="Test Slider" class="Slide (strict)"("Visible"=FALSE) -> ()  [unwired: 2 in, 2 out]
              }
              frame "Exposure Priority  **" {
                n207 = Index Array(array=w354, index=3) -> (element=w355:cluster{string[]})
                n208 = call <vilib>:"NT Read String.vi"("Name"=w357) -> ("String"=w356:string)  [unwired: 9 in, 1 out]
                n209 = Unbundle(w355) -> (w351:string[])
                n210 = Match First String(2:w351, 3:w356) -> (0:w352:i32)  [unwired: 1 out]
                n211 = property on="Test Ring" class="Ring (strict)"("Value"=w352, "Strings []"=w351) -> ()  [unwired: 2 in, 2 out]
                n212 = property on="Test Ring" class="Ring (strict)"("Visible"=TRUE) -> ()  [unwired: 2 in, 2 out]
                n213 = property on="Test Slider" class="Slide (strict)"("Visible"=FALSE) -> ()  [unwired: 2 in, 2 out]
              }
              frame "Color Enable  **" {
                n214 = Index Array(array=w363, index=4) -> (element=w364:cluster{string[]})
                n215 = call <vilib>:"NT Read String.vi"("Name"=w366) -> ("String"=w365:string)  [unwired: 9 in, 1 out]
                n216 = Unbundle(w364) -> (w360:string[])
                n217 = Match First String(2:w360, 3:w365) -> (0:w361:i32)  [unwired: 1 out]
                n218 = property on="Test Ring" class="Ring (strict)"("Value"=w361, "Strings []"=w360) -> ()  [unwired: 2 in, 2 out]
                n219 = property on="Test Ring" class="Ring (strict)"("Visible"=TRUE) -> ()  [unwired: 2 in, 2 out]
                n220 = property on="Test Slider" class="Slide (strict)"("Visible"=FALSE) -> ()  [unwired: 2 in, 2 out]
              }
              frame Default {
                n221 = property on="Test Ring" class="Ring (strict)"("Visible"=FALSE) -> ()  [unwired: 2 in, 2 out]
                n222 = property on="Test Slider" class="Slide (strict)"("Visible"=FALSE) -> ()  [unwired: 2 in, 2 out]
              }
              frame "Brightness  **", "Color Level  **", "Compression  **", "FPS  **", "Sharpness  **" {
                n223 = call <vilib>:"NT Read Number.vi"("Name"=w372) -> ("Numeric"=w371:dbl)  [unwired: 9 in, 1 out]
                n224 = local write "Test Slider"(w371) -> ()
                n225 = property on="Test Slider" class="Slide (strict)"("Visible"=TRUE, "Scale.Maximum"=100.0 ("Scale.Range:Maximum")) -> ()  [unwired: 2 in, 2 out]
                n226 = property on="Test Ring" class="Ring (strict)"("Visible"=FALSE) -> ()  [unwired: 2 in, 2 out]
              }
            }
          }
        }
        n227 = property on="Progress" class="Clust (strict)"("Visible"=FALSE) -> ()  [unwired: 2 in, 2 out]
      }
      event "Test Name": Mouse Enter {
        # "Populate the ring with the list of tests"
        n228 = event-data() -> ()  [unwired: 1 in, 1 out]
        n229 = call <vilib>:"NT Read String Array.vi"("Name"="TestMode/TestList") -> ("String Array"=w380:string[])  [unwired: 9 in, 1 out]
        n230 = Build Array (concatenate)("Select the test to run...", w380) -> (w379:string[])
        n231 = property on="Test Name" class="Ring (strict)"("Strings []"=w379) -> ()  [unwired: 2 in, 2 out]
      }
      event "Test Name": Value Change {
        w382 = FALSE ("Visible")
        # "Tell the robot the test name to run"
        n232 = event-data() -> ("NewVal"=w386:u16)  [unwired: 1 in]
        n233 = property on="Test Name" class="Ring (strict)"() -> ("Strings []"=w387:string[])  [unwired: 2 in, 2 out]
        n234 = local write "Progress"(T5 {"Test Progress"=0, "Test Progress Text"=""} ("Progress")) -> ()
        n235 = Index Array(array=w387, index=w386) -> (element=w385:string)
        n236 = call <vilib>:"NT Write String.vi"("String"=w385, "Name"="TestMode/TestName") -> ()  [unwired: 9 in, 1 out]
        n237 = property on="Progress" class="Clust (strict)"("Visible"=TRUE) -> ()  [unwired: 2 in, 2 out]
        n238 = property on="Motor" class="Clust (strict)"("Visible"=w382) -> ()  [unwired: 2 in, 2 out]
        n239 = property on="Test Slider" class="Slide (strict)"("Visible"=w382) -> ()  [unwired: 2 in, 2 out]
        n240 = property on="On/Off" class="Bool (strict)"("Visible"=w382) -> ()  [unwired: 2 in, 2 out]
        n241 = property on="Rev/Fwd" class="Clust (strict)"("Visible"=w382) -> ()  [unwired: 2 in, 2 out]
        n242 = property on="Test Ring" class="Ring (strict)"("Visible"=w382) -> ()  [unwired: 2 in, 2 out]
      }
      event "Select Auto": Mouse Enter {
        # "Populate the combo box with the list of autonomous options"
        n243 = event-data() -> ()  [unwired: 1 in, 1 out]
        n244 = call <vilib>:"NT Read String Array.vi"("Name"="Auto List") -> ("String Array"=w389:string[])  [unwired: 9 in, 1 out]
        n245 = property on="Select Auto" class="CmbBox"("Strings[]"=w389) -> ()  [unwired: 2 in, 2 out]
      }
      event "Select Auto": Value Change {
        # "User modified the Auto Selection. Write to NT variable so robot knows."
        n246 = event-data() -> ("NewVal"=w392:string)  [unwired: 1 in]
        n247 = call <vilib>:"NT Write String.vi"("String"=w392, "Name"="Auto Selector") -> ()  [unwired: 9 in, 1 out]
      }
      event "Command Selection": Value Change {
        # "Get the params and show in table"
        n248 = event-data() -> ("NewVal"=w398:i32)  [unwired: 1 in]
        n249 = property on="Command Selection" class="MCListbox (strict)"() -> ("ItemNames"=w396:string[][])  [unwired: 2 in, 2 out]
        n250 = call <vilib>:"WPI_DashboardUpdate Command Params.vi"("NewVal"=w398, "Commands"=w396, "Param Tbl"=w397) -> ()  [unwired: 8 in, 1 out]
      }
      event "Execute Command": Value Change {
        # "Started one, Unique ID holds\nresponse"
        n251 = event-data() -> ()  [unwired: 1 in, 1 out]
        n252 = property on="Command Selection" class="MCListbox (strict)"() -> ("ItemNames"=w409:string[][])  [unwired: 2 in, 2 out]
        n253 = Index Array(array=w409, index (row)="Command Selection", index (col)=0) -> (element=w407:string)
        n254 = call <vilib>:"Invoke Commands.vi"("Command Params"="Command Params", "Function Name"=w407) -> ("Params"=w403:u8, "Started"=w402:bool)  [unwired: 7 in, 1 out]
        n255 = Array Subset(array="Command Params", length (row)=w403) -> (w404:string[][])  [unwired: 3 in]
        n256 = Select(t="Executing" ("Cmd Status"), s=w402, f="" ("Cmd Status")) -> (s? t:f=→"Cmd Status":string)
      }
      event "Command Selection": Double Click {
        n257 = event-data() -> ("Row"=w417:i32)  [unwired: 1 in]
        n258 = property on="Command Selection" class="MCListbox (strict)"() -> ("ItemNames"=w420:string[][])  [unwired: 2 in, 2 out]
        n259 = local read "Command Params"() -> (w416:string[][])
        n260 = Index Array(array=w420, index (row)=w417, index (col)=0) -> (element=w418:string)
        n261 = call <vilib>:"Invoke Commands.vi"("Command Params"=w416, "Function Name"=w418) -> ("Params"=w415:u8, "Started"=w410:bool)  [unwired: 7 in, 1 out]
        n262 = Array Subset(array=w416, length (row)=w415) -> (w414:string[][])  [unwired: 3 in]
        n263 = Select(t="Executing" ("Cmd Status"), s=w410, f="" ("Cmd Status")) -> (s? t:f=w411:string)
        n264 = local write "Cmd Status"(w411) -> ()
      }
      event "CheckList": Double Click {
        # "Shift clears all"
        # "Update symbols on the listbox"
        n265 = event-data() -> ("PlatMods.Shift"=w422:bool, "Row"=w424:i32)  [unwired: 1 in]
        n266 = case shown="False" w422 {
          tunnel: w424 -> [w428 _]
          tunnel: 1 -> [w427 _]
          frame False {
            n267 = property on="CheckList" class="LstBox (strict)"() -> ("Item Symbols"=w426:i32[])  [unwired: 2 in, 2 out]
            n268 = Replace Array Subset(array=w426, new element=w427, index=w428) -> (w425:i32[])
            n269 = property on="CheckList" class="LstBox (strict)"("Item Symbols"=w425) -> ()  [unwired: 2 in, 2 out]
          }
          frame True {
            w429 = 0 ("Top Row")
            n270 = property on="CheckList" class="LstBox (strict)"() -> ("Number of Rows"=w431:u32)  [unwired: 2 in, 2 out]
            n271 = Initialize Array(0, w431) -> (w430:i32[])
            n272 = property on="CheckList" class="LstBox (strict)"("Top Row"=w429, "Value"=w429, "Item Symbols"=w430) -> ()  [unwired: 2 in, 2 out]
          }
        }
      }
      event "CheckList": Key Down {
        # "Update symbols on the listbox\nLeft and right keys check and uncheck"
        n273 = event-data() -> ("VKey"=w435:T20)  [unwired: 1 in]
        n274 = case shown="\"Left\", \"Right\"" w435 {
          selector: w435 -> [w440 _]
          tunnel: eventvkey."Left" ("VKey") -> [w438 _]
          frame "Left", "Right" {
            n275 = Equal?(x=w438, y=w440) -> (x = y?=w439:bool)
            n276 = Select(t=0, s=w439, f=1) -> (s? t:f=w441:i32)
            n277 = property on="CheckList" class="LstBox (strict)"() -> ("Item Symbols"=w444:i32[])  [unwired: 2 in, 2 out]
            n278 = Replace Array Subset(array=w444, new element=w441, index="CheckList") -> (w443:i32[])
            n279 = property on="CheckList" class="LstBox (strict)"("Item Symbols"=w443) -> ()  [unwired: 2 in, 2 out]
          }
          frame Default {
          }
        }
      }
      event "Motor.Enable": Value Change {
        # "When the test mode otor enable helper is set, update that\ntree row item's value"
        n280 = event-data() -> ("NewVal"=w450:bool)  [unwired: 1 in]
        n281 = Unbundle("Motor") -> ("Value"=w449:dbl)  [unwired: 1 out]
        n282 = Select(t=w449, s=w450, f=0.0) -> (s? t:f=w447:dbl)
        n283 = call <vilib>:"NT Write Number.vi"("Numeric"=w447, "Name"=w446) -> ()  [unwired: 9 in, 1 out]
      }
      event "Test Slider": Value Change {
        # "When the test mode slider helper is set, update that\ntree row item's value"
        n284 = event-data() -> ("NewVal"=w453:dbl)  [unwired: 1 in]
        n285 = call <vilib>:"NT Write Number.vi"("Numeric"=w453, "Name"=w454) -> ()  [unwired: 9 in, 1 out]
      }
      event "On/Off": Value Change {
        # "When the test mode on/off helper value is set, update that\ntree row item's value"
        n286 = event-data() -> ("NewVal"=w458:bool)  [unwired: 1 in]
        n287 = Boolean To (0,1)(Boolean=w458) -> (0, 1=w457:i16)
        n288 = call <vilib>:"NT Write Number.vi"("Numeric"=w457, "Name"=w456) -> ()  [unwired: 9 in, 1 out]
      }
      event "Rev/Fwd": Value Change {
        # "When the test mode helper value for relays is set, update that\ntree row item's value"
        n289 = event-data() -> ("NewVal.Forward"=w466:bool, "NewVal.Reverse"=w465:bool)  [unwired: 1 in]
        n290 = Boolean To (0,1)(Boolean=w466) -> (0, 1=w462:i16)
        n291 = Boolean To (0,1)(Boolean=w465) -> (0, 1=w464:i16)
        n292 = Negate(x=w464) -> (-x=w463:i16)
        n293 = Add(x=w462, y=w463) -> (x+y=w461:i16)
        n294 = call <vilib>:"NT Write Number.vi"("Numeric"=w461, "Name"=w460) -> ()  [unwired: 9 in, 1 out]
      }
      event "Test Ring": Value Change {
        # "When a test mode helper value is selected from the ring,\nset the tree item's variable to the string value"
        n295 = event-data() -> ("NewVal"=w470:u16)  [unwired: 1 in]
        n296 = property on="Test Ring" class="Ring (strict)"() -> ("Strings []"=w471:string[])  [unwired: 2 in, 2 out]
        n297 = Index Array(array=w471, index=w470) -> (element=w469:string)
        n298 = call <vilib>:"NT Write String.vi"("String"=w469, "Name"=w468) -> ()  [unwired: 9 in, 1 out]
      }
      event "Rec Mode": Value Change {
        # "Update globals for recording mode and path to read log from.\nClear when logging and let NetworkTables set path for vision to\nuse."
        n299 = event-data() -> ("NewVal"=w480:enum32{"Stop", "Record", "Playback"})  [unwired: 1 in]
        n300 = global write "WPI_DashboardLogging Global.vi" "Logging Filename"(path "") -> ()
        n301 = global write "WPI_DashboardLogging Global.vi" "Recording"(w480) -> ()
        n302 = case shown="\"Playback\"" w480 {
          tunnel: w479 -> [_ w482 w489]
          tunnel: [_ _ w488] -> w477
          tunnel: [_ _ w487] -> _
          tunnel: w475 -> [_ _ w485]
          tunnel: cluster{i32, i32} {-250, 170} -> [_ _ w484]
          tunnel: w473 -> [_ _ w483]
          frame Default {
          }
          frame "Stop", "Record" {
            # "Place Window too"
            n303 = invoke class="VI" method="FP.Close"(reference=w482) -> (reference out=w481:refnum<vi>)  [unwired: 2 in, 2 out]
            n304 = invoke class="VI" method="Abort VI"(reference=w481) -> ()  [unwired: 2 in, 3 out]
          }
          frame "Playback" {
            n305 = call "Open Playback Panel.vi"("Offset"=w484, "DB VI Ref"=w485, "Playback in"=w489) -> ("Playback out"=w486:refnum<vi>)  [unwired: 8 in]
            n306 = register-events(w486, w483) -> (reference out=w488:refnum<event-registration>, error out=w487:errorcluster)  [unwired: 2 in]
          }
        }
        n307 = call <vilib>:"WPI_DashboardNT Log FieldName Cache.vi"("Operation"=enum16{"Lookup/Add", "Index", "Clear"}."Clear") -> ()  [unwired: 8 in, 3 out]
      }
      event Panel Close {
        w491 = enum32{"Stop", "Record", "Playback"}."Stop" ("Rec Mode")
        # "Playback window has been closed, abort"
        n308 = event-data() -> ()  [unwired: 1 in, 4 out]
        n309 = local write "Rec Mode"(w491) -> ()
        n310 = global write "WPI_DashboardLogging Global.vi" "Recording"(w491) -> ()
      }
      event Panel Close {
        # "Abort playback window and ourself"
        n311 = event-data() -> ()  [unwired: 1 in, 4 out]
        n312 = invoke class="VI" method="FP.Close"(reference=w495) -> (reference out=w494:refnum<vi>)  [unwired: 2 in, 2 out]
        n313 = invoke class="VI" method="Abort VI"(reference=w494) -> (error out=w493:errorcluster)  [unwired: 2 in, 2 out]
        n314 = invoke class="VI" method="Abort VI"(error in=w493) -> ()  [unwired: 2 in, 3 out]
      }
      event User Event {
        n315 = event-data() -> ("IDs"=w502:cluster{"RPC field ID":u16, "Unique ID":u16}, "String"=w501:string)  [unwired: 1 in]
        n316 = Bundle("IDs"=w502, "String"=w501) -> (w500:T10)  [unwired: 1 in]
        n317 = call <vilib>:"Retrieve RPC Response.vi"("RPC Response"=w500) -> ("Output"=w498:string[][])  [unwired: 10 in]
        n318 = Build Array (concatenate)(w496, w498) -> (w497:string[][])
        n319 = local write "Command Params"(w497) -> ()
        n320 = local write "Cmd Status"("" ("Cmd Status")) -> ()
      }
      event "Tree": Double Click {
        n321 = event-data() -> ("PlatMods"=w508:T23, "Tag"=w505:string)  [unwired: 1 in]
        n322 = Unbundle(w508) -> ("Shift"=w507:bool)  [unwired: 4 out]
        n323 = String Subset(string=w505, length (rest)=1 ("length (rest)")) -> (substring=w504:string)  [unwired: 1 in]
        n324 = Not(x=w507) -> (.not. x?=w506:bool)
        n325 = case shown="\"/\"" w504 {
          tunnel: w505 -> [_ w511]
          tunnel: w506 -> [_ w510]
          frame Default {
          }
          frame "/" {
            n326 = call <vilib>:"NT Update Persistence.vi"("Persistence"=w510, "Name"=w511) -> ()  [unwired: 9 in, 1 out]
          }
        }
      }
    }
  }
  n327 = while {
    tunnel: w61 -> [w513]
    i -> [w516]
    stop <- FALSE stop-if-true
    n328 = Wait (ms)(milliseconds to wait=u32 100) -> ()  [unwired: 1 out]
    n329 = case shown="\"Playback\"" "Rec Mode" {
      tunnel: w516 -> [_ _ w531]
      tunnel: [u32 2829099 ("Base Color") u32 11141120 ("Target Color") w520] -> w512
      frame "Stop", Default {
        # "Reset the color, extra updates don't cost much"
      }
      frame "Record" {
      }
      frame "Playback" {
        # "Playback"
        n330 = Quotient & Remainder(x=w531, y=u32 50 ("milliseconds to wait")) -> (x-y*floor(x/y)=w527:u32)  [unwired: 1 out]
        n331 = Divide(x=w527, y=u32 50 ("milliseconds to wait")) -> (x/y=w524:dbl)
        n332 = Multiply(x=6.283185307179586, y=w524) -> (x*y=w529:dbl)
        n333 = Sine(x=w529) -> (sin(x)=w528:dbl)
        n334 = Absolute Value(x=w528) -> (abs(x)=w521:dbl)
        n335 = call "Interpolate RGB Color.vi"("Proportion"=w521, "Target Color"=u32 30976, "Base Color"=u32 2829099) -> ("Result Color"=w520:u32)  [unwired: 8 in]
      }
    }
    n336 = property class="Pane"(reference=w513, "PaneColor"=w512) -> ()  [unwired: 1 in, 2 out]
  }
  n337 = property on="On/Off" class="Bool (strict)"("Visible"=w34) -> ()  [unwired: 2 in, 2 out]
  n338 = property on="Motor" class="Clust (strict)"("Visible"=w34) -> ()  [unwired: 2 in, 2 out]
  n339 = property on="Progress" class="Clust (strict)"("Visible"=w34) -> ()  [unwired: 2 in, 2 out]
  n340 = property on="Test Ring" class="Ring (strict)"("Visible"=w34) -> ()  [unwired: 2 in, 2 out]
  n341 = property on="Rev/Fwd" class="Clust (strict)"("Visible"=w34) -> ()  [unwired: 2 in, 2 out]
  n342 = while {
    tunnel: u16 1741 ("timeout ms (25000)") -> [w533]
    stop <- FALSE stop-if-true
    n343 = TCP Create Listener(10:w533) -> (0:w532:errorcluster, 3:w534:refnum<k5>)  [unwired: 4 in, 1 out]
    n344 = case shown="No Error" w532 {
      selector: w532 -> [w536 _]
      tunnel: w534 -> [w537 _]
      frame No Error {
        n345 = while {
          tunnel: w537 -> [w540]
          tunnel: w536 -> [w539]
          stop <- FALSE stop-if-true
          n346 = TCP Wait On Listener(8:w539, 11:w540) -> (0:w541:errorcluster, 4:w542:refnum<k5>)  [unwired: 2 in, 3 out]
          n347 = local write "TCP"(w542) -> ()
          n348 = case shown="No Error" w541 {
            frame No Error {
            }
            frame Error {
              n349 = Wait (ms)(milliseconds to wait=u32 1000) -> ()  [unwired: 1 out]
            }
          }
        }
      }
      frame Error {
        n350 = Wait (ms)(milliseconds to wait=u32 1000) -> ()  [unwired: 1 out]
      }
    }
  }
  n351 = local write "Command Selection"(u16 0 ("milliseconds to wait")) -> ()
  n352 = local write "Command Params"(string[][] [] ("Command Params")) -> ()
  n353 = global write "WPI_DashboardLogging Global.vi" "Recording"(w55) -> ()
  n354 = local write "Rec Mode"(w55) -> ()
  n355 = call <vilib>:"NT Write String.vi"("String"="Select Auto", "Name"="Auto Selector") -> ()  [unwired: 9 in, 1 out]
